vi "test_sub_VIs.vi"() -> ()   [LabVIEW 2024]
panel:
  in  "Degrees":dbl
  in  "Motor \"Name\"":string="1"
  in  "VISA resource name":refnum<visa-resource-name>="COM3"
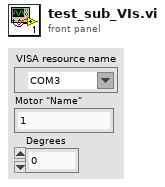
[diagram p1: front panel]
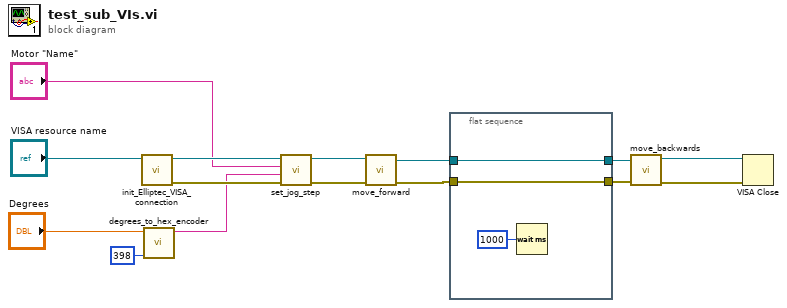
[diagram p0: block diagram]
diagram:
  n1 = call "init_Elliptec_VISA_connection.vi"("VISA resource name"="VISA resource name") -> ("error out"=w13:errorcluster, "VISA resource name out"=w14:refnum<visa-resource-name>)  [unwired: 9 in]
  n2 = call "degrees_to_hex_encoder.vi"("Encoder Pulses per Degree"=398, "Degrees"="Degrees") -> ("hex integer string"=w8:string)  [unwired: 8 in, 1 out]
  n3 = call "set_jog_step.vi"("error in (no error)"=w13, "Encoder Pulses"=w8, "Motor \"Name\""="Motor \"Name\"", "VISA resource name"=w14) -> ("error out"=w10:errorcluster, "VISA resource name out"=w11:refnum<visa-resource-name>)  [unwired: 5 in]
  n4 = call "move_forward.vi"("error in (no error)"=w10, "VISA resource name"=w11) -> ("error out"=w3:errorcluster, "VISA resource name out"=w5:refnum<visa-resource-name>)  [unwired: 8 in]
  n5 = flat-sequence {
    tunnel: [w18] -> w6
    tunnel: w5 -> [w18]
    tunnel: [w17] -> w4
    tunnel: w3 -> [w17]
    frame #0 {
      n6 = Wait (ms)(milliseconds to wait=u32 1000) -> ()  [unwired: 1 out]
    }
  }
  n7 = call "move_backwards.vi"("error in (no error)"=w4, "VISA resource name"=w6) -> ("error out"=w1:errorcluster, "VISA resource name out"=w2:refnum<visa-resource-name>)  [unwired: 8 in]
  n8 = VISA Close(VISA resource name=w2, error in (no error)=w1) -> ()  [unwired: 1 out]
